vi "Process_InOutData.vi"(7 "Real":dbl=3.0, 8 "InOutBool":dbl[](array[numeric]), 9 "TimeData":dbl[](array[numeric]), 10 "f0_f9Phase":dbl[][](array[numeric]), 11 "f0_f9Mag":dbl[][](array[numeric]) format="%#_2p") -> (0 "SNR":dbl[][](array[numeric]), 1 "Betas":dbl[][](array[numeric]) format="%#_2p", 2 "DriftTerms":dbl[][](array[numeric]), 3 "Yhat":dbl[][](array[numeric]) format="%#_2p", 4 "Noise":dbl[][](array[numeric]), 6 "nHat":dbl[][](array[numeric]))   [LabVIEW 2021]
panel:
  out "nHat2":dbl[](graph)
  out "Sample Out2":dbl[](graph)
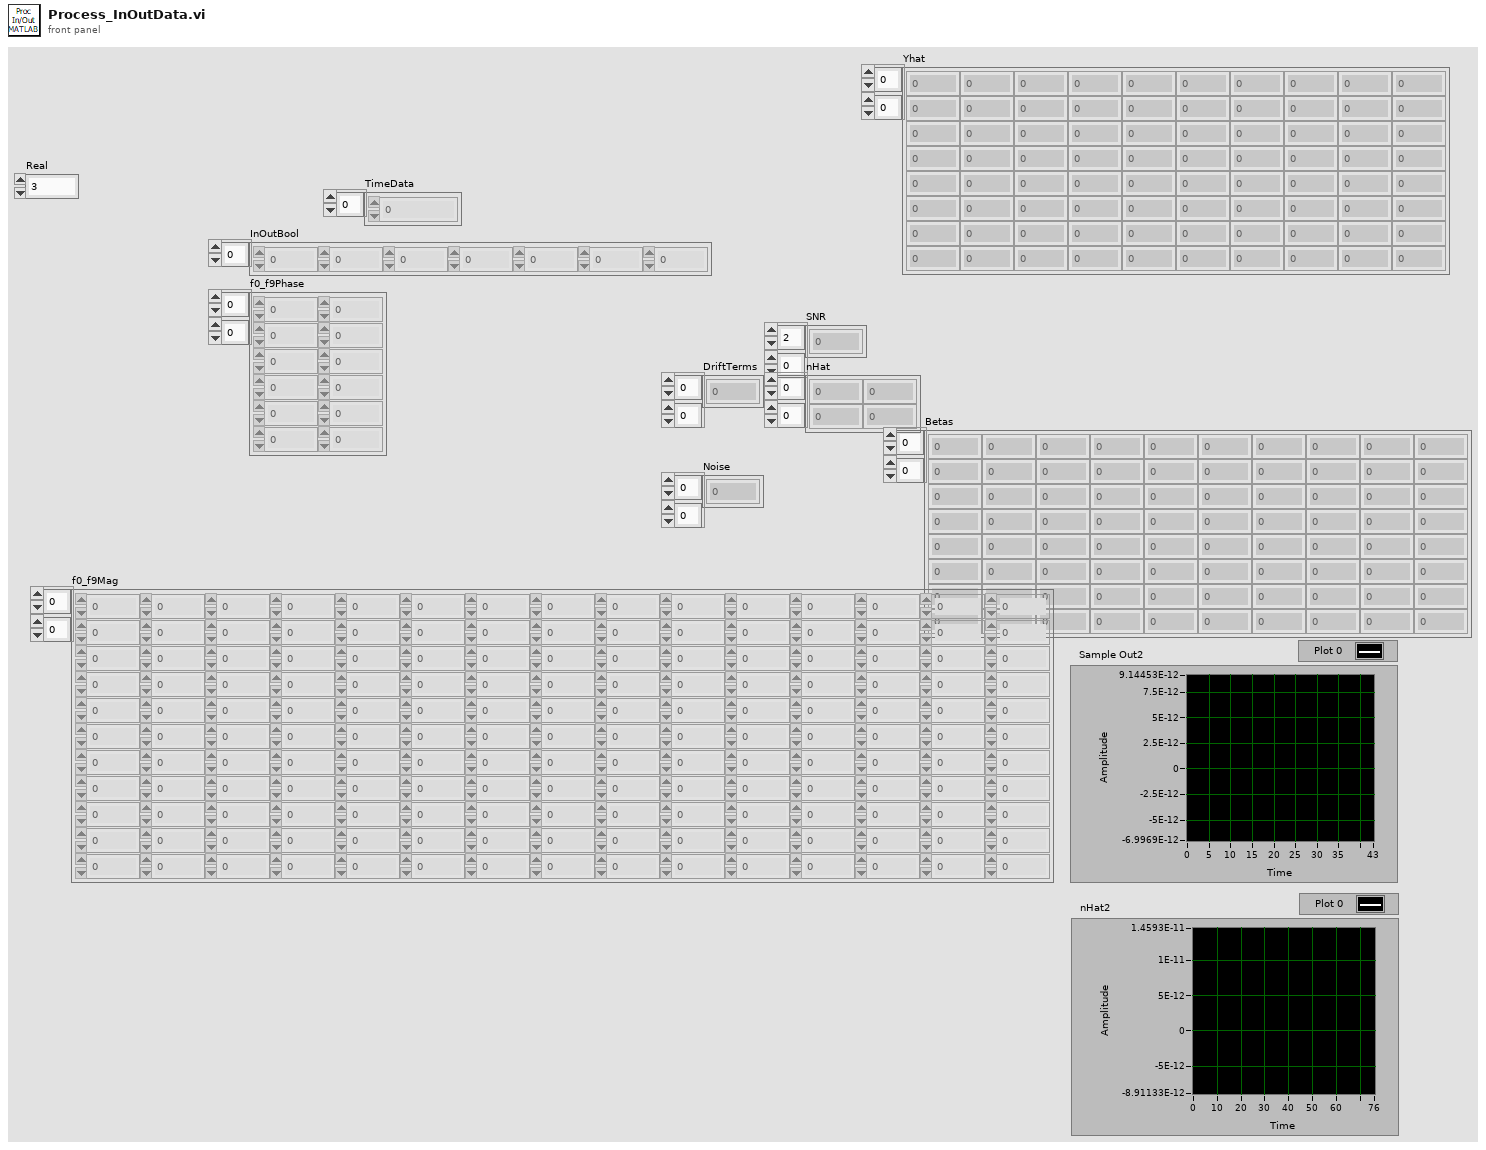
[diagram p1: front panel]
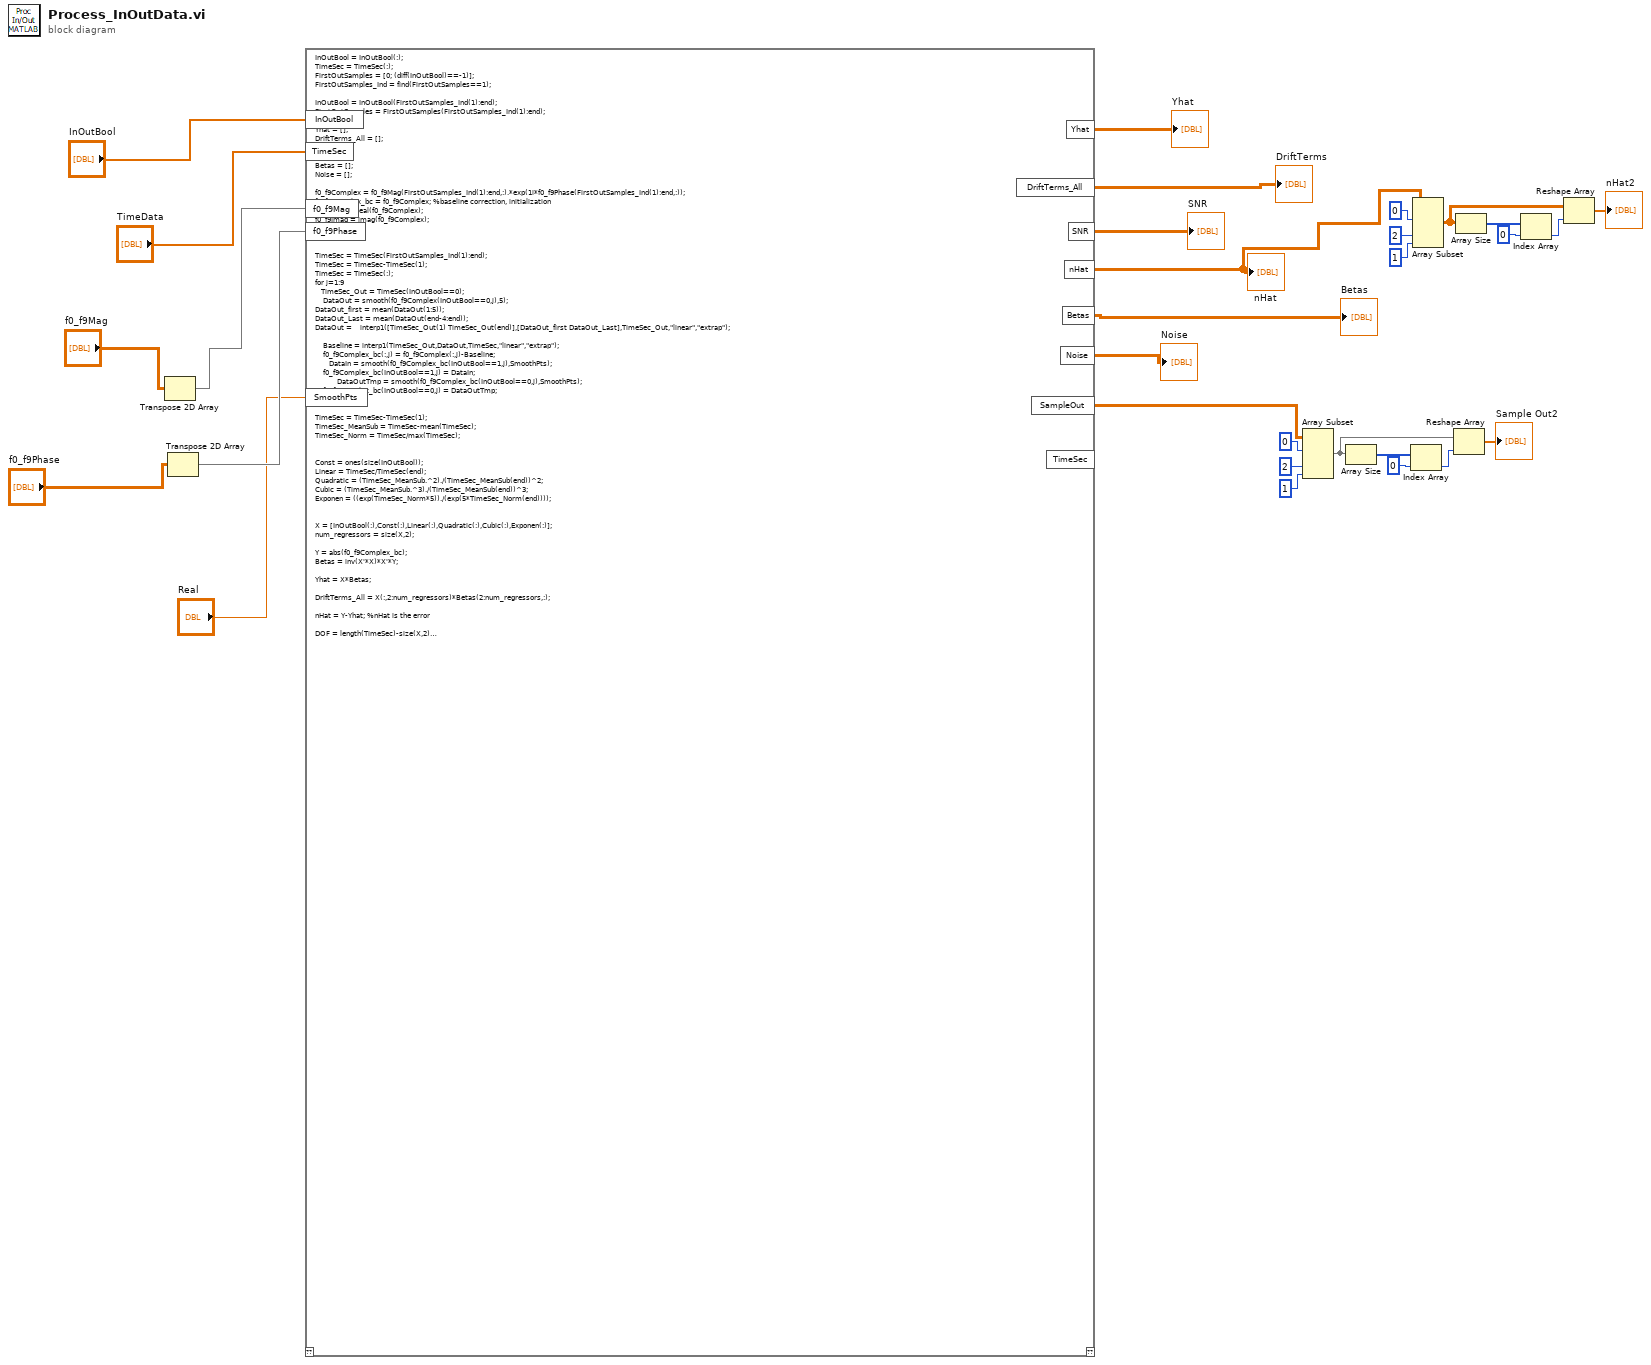
[diagram p0: block diagram]
diagram:
  n1 = Transpose 2D Array(2D array="f0_f9Mag") -> (transposed array=w20:dbl[][])
  n2 = Transpose 2D Array(2D array="f0_f9Phase") -> (transposed array=w22:dbl[][])
  n3 = script code="InOutBool = InOutBool(:);\nTimeSec = TimeSec(:);\nFirstOutSamples = [0; (diff(InOutBool)==-1)];\nFirstOutSamples_Ind = find(FirstOutSamples==1);\n\nInOutBool = InOutBool(FirstOutSamples_Ind(1):end);\nFirstOutSamples = FirstOutSamples(FirstOutSamples_Ind(1):end);\n\nYhat = [];\nDriftTerms_All = [];\nSNR = [];\nnHat = [];\nBetas = [];\nNoise = [];\n\nf0_f9Complex = f0_f9Mag(FirstOutSamples_Ind(1):end,:).*exp(1i*f0_f9Phase(FirstOutSamples_Ind(1):end,:));\nf0_f9Complex_bc = f0_f9Complex; %baseline correction, initialization\nf0_f9Real = real(f0_f9Complex);\nf0_f9Imag = imag(f0_f9Complex);\n\n\n\nTimeSec = TimeSec(FirstOutSamples_Ind(1):end);\nTimeSec = TimeSec-TimeSec(1);\nTimeSec = TimeSec(:);\nfor j=1:9\n   TimeSec_Out = TimeSec(InOutBool==0);\n    DataOut = smooth(f0_f9Complex(InOutBool==0,j),5);\nDataOut_first = mean(DataOut(1:5));\nDataOut_Last = mean(DataOut(end-4:end));\nDataOut =    interp1([TimeSec_Out(1) TimeSec_Out(end)],[DataOut_first DataOut_Last],TimeSec_Out,\"linear\",\"extrap\");\n\n    Baseline = interp1(TimeSec_Out,DataOut,TimeSec,\"linear\",\"extrap\");\n    f0_f9Complex_bc(:,j) = f0_f9Complex(:,j)-Baseline;\n       DataIn = smooth(f0_f9Complex_bc(InOutBool==1,j),SmoothPts);\n    f0_f9Complex_bc(InOutBool==1,j) = DataIn; \n           DataOutTmp = smooth(f0_f9Complex_bc(InOutBool==0,j),SmoothPts);\n    f0_f9Complex_bc(InOutBool==0,j) = DataOutTmp; \nend\n\nTimeSec = TimeSec-TimeSec(1);\nTimeSec_MeanSub = TimeSec-mean(TimeSec);\nTimeSec_Norm = TimeSec/max(TimeSec);\n\n\nConst = ones(size(InOutBool));\nLinear = TimeSec/TimeSec(end);\nQuadratic = (TimeSec_MeanSub.^2)./(TimeSec_MeanSub(end))^2;\nCubic = (TimeSec_MeanSub.^3)./(TimeSec_MeanSub(end))^3;\nExponen = ((exp(TimeSec_Norm*5))./(exp(5*TimeSec_Norm(end))));\n\n\nX = [InOutBool(:),Const(:),Linear(:),Quadratic(:),Cubic(:),Exponen(:)];\nnum_regressors = size(X,2);\n\nY = abs(f0_f9Complex_bc);\nBetas = inv(X'*X)*X'*Y;\n\nYhat = X*Betas;\n\nDriftTerms_All = X(:,2:num_regressors)*Betas(2:num_regressors,:);\n\nnHat = Y-Yhat; %nHat is the error\n\nDOF = length(TimeSec)-size(X,2);\nResidualVariance = diag(nHat'*nHat)/DOF; % Mean Square Error\n\nC = [1 0 0 0 0 0];\nGamma = C*Betas; % Gamma = Betas for Activation regressor only\n\nActivationReg_Energy = C*inv(X'*X)*C';\nContrastVariance = ActivationReg_Energy*ResidualVariance; % error^2/Power\ntDOF = Gamma./sqrt(ContrastVariance); % coefficients/sqrt(noise^2/Power) --> how far from mean relative to noise\n\n\n\nSampleOut = nHat(InOutBool==0,:);\n\nNoise = abs(std(nHat(InOutBool==0,:),0,1)); % \n\n\nGamma_norm = Gamma/sqrt(ActivationReg_Energy*DOF);\n%         CNR = Gamma_norm./(Noise);\nSNR = Gamma./(Noise);  \nSNR = abs(SNR(:));"("InOutBool"="InOutBool", "TimeSec"="TimeData", "f0_f9Mag"=w20, "f0_f9Phase"=w22, "SmoothPts"="Real") -> ("Yhat"=→"Yhat":dbl[][], "DriftTerms_All"=→"DriftTerms":dbl[][], "SNR"=→"SNR":dbl[][], "nHat"=w2:dbl[][], "Betas"=→"Betas":dbl[][], "Noise"=→"Noise":dbl[][], "SampleOut"=w16:dbl[][])  [unwired: 1 in, 2 out]
  "nHat" <- w2
  n4 = Array Subset(array=w16, index (row)=0 ("index"), index (col)=2 ("index"), length (col)=1 ("length")) -> (w13:dbl[][])  [unwired: 1 in]
  n5 = Array Size(array=w13) -> (size(s)=w14:i32[])
  n6 = Index Array(array=w14, index=0) -> (element=w11:i32)
  n7 = Array Subset(array=w2, index (row)=0 ("index"), index (col)=2 ("index"), length (col)=1 ("length")) -> (w8:dbl[][])  [unwired: 1 in]
  n8 = Reshape Array(w13, w11) -> (→"Sample Out2":dbl[])
  n9 = Array Size(array=w8) -> (size(s)=w7:i32[])
  n10 = Index Array(array=w7, index=0) -> (element=w10:i32)
  n11 = Reshape Array(w8, w10) -> (→"nHat2":dbl[])
